vi "HandleSharedVariablTesting.vi"(0 "reference in":refnum<class "Stand.lvclass">, 11 "error in (no error)":errorcluster) -> (4 "reference out":refnum<class "Stand.lvclass">, 15 "error out":errorcluster)   [LabVIEW 2019, in "Stand.lvclass"]
uses:
  Stand.lvclass
  Stand.lvclass/Stand.ctl
  Sig_DO_Simple_class/Sig_DO_Simple.lvclass/Sig_DO_Simple.ctl
  Proccess_class/Proccess.lvclass/Proccess.ctl
  Sig_AO_class/Sig_AO.lvclass/Sig_AO.ctl
  Logger_class/Logger.lvclass/Logger.ctl
  Sig_DO_Simple_class/private/write_do_to_db.vi
  Sig_AO_class/private/WriteToDb.vi
  Proccess_class/Read TagName.vi
  Proccess_class/Read Logger.vi
  Logger_class/Enqueue Signal.vi
  Sig_DO_Simple_class/Sig_DO_Simple.lvclass
  D:/H4000/src/Proccess_class/Proccess.lvclass
  Sig_AO_class/Sig_AO.lvclass
  Logger_class/WriteEvent.vi
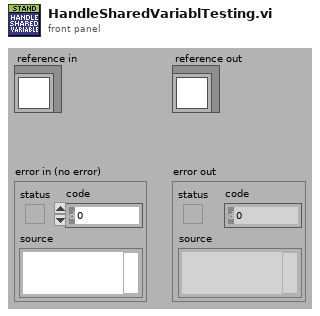
[diagram p1: front panel]
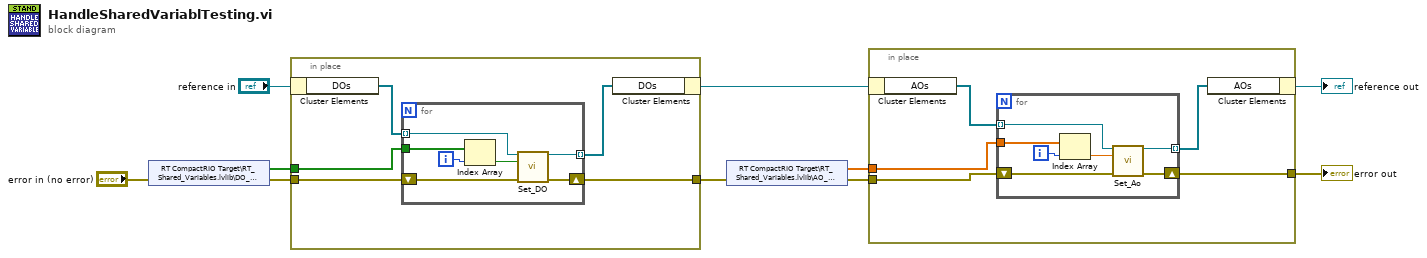
[diagram p0: block diagram]
diagram:
  n1 = shared-variable "RT CompactRIO Target\\RT_Shared_Variables.lvlib\\DO_ARRAY_IN"(error in="error in (no error)") -> (w10:bool[], error out=w9:errorcluster)
  n2 = in-place {
    in-place-border: w10 -> [w15]
    in-place-border: w9 -> [w14]
    in-place-border: [w13] -> w3
    n3 = in-place-cluster #1("reference in") -> ("DOs"=w12:refnum<class "Sig_DO_Simple.lvclass">[])
    n4 = for {
      tunnel: w15 -> [w22]
      tunnel: [w17] -> w11 mode=indexing
      shift-right: [w18] -> w13
      shift-left: w14 -> [w19]
      tunnel: w12 -> [w16] mode=indexing
      i -> [w21]
      n5 = Index Array(array=w22, index=w21) -> (element=w20:bool)
      n6 = call "Set_DO.vi"("reference in"=w16, "DO"=w20, "error in (no error)"=w19) -> ("reference out"=w17:refnum<class "Sig_DO_Simple.lvclass">, "error out"=w18:errorcluster)  [unwired: 11 in]
    }
    n7 = in-place-cluster #1("DOs"=w11) -> (w6:refnum<class "Stand.lvclass">)
  }
  n8 = shared-variable "RT CompactRIO Target\\RT_Shared_Variables.lvlib\\AO_ARRAY_IN"(error in=w3) -> (w1:dbl[], error out=w2:errorcluster)
  n9 = in-place {
    in-place-border: w1 -> [w27]
    in-place-border: w2 -> [w26]
    in-place-border: [w25] -> w4
    n10 = in-place-cluster #2(w6) -> ("AOs"=w24:refnum<class "Sig_AO.lvclass">[])
    n11 = for {
      tunnel: w27 -> [w34]
      tunnel: [w29] -> w23 mode=indexing
      shift-right: [w30] -> w25
      shift-left: w26 -> [w31]
      tunnel: w24 -> [w28] mode=indexing
      i -> [w33]
      n12 = Index Array(array=w34, index=w33) -> (element=w32:dbl)
      n13 = call "Set_Ao.vi"("reference in"=w28, "AO"=w32, "error in (no error)"=w31) -> ("reference out"=w29:refnum<class "Sig_AO.lvclass">, "error out"=w30:errorcluster)  [unwired: 11 in]
    }
    n14 = in-place-cluster #2("AOs"=w23) -> (→"reference out":refnum<class "Stand.lvclass">)
  }
  "error out" <- w4
